vi "OperateDatabase.vi"(8 "error in (no error)":errorcluster, 10 "Person in":refnum<class "Person.lvclass">, 11 "State_Visitor in":refnum<class "State_Visitor.lvclass">) -> (0 "error out":errorcluster, 2 "Person out":refnum<class "Person.lvclass">, 3 "State_Visitor out":refnum<class "State_Visitor.lvclass">)   [LabVIEW 2014, in "State_Visitor.lvclass"]
uses:
  State_Visitor.lvclass
  Person_Class/Person.lvclass
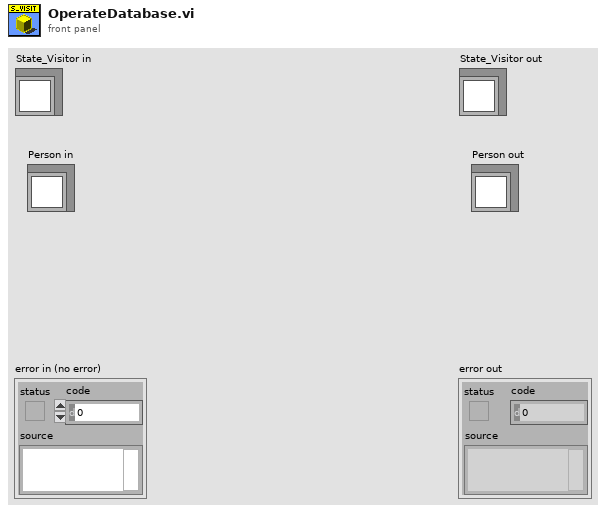
[diagram p1: front panel]
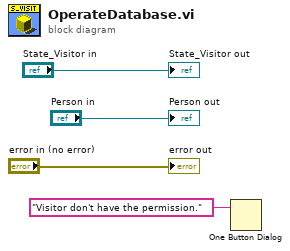
[diagram p0: block diagram]
diagram:
  n1 = One Button Dialog(message="Visitor don't have the permission.") -> ()  [unwired: 1 in, 1 out]
  "error out" <- "error in (no error)"
  "State_Visitor out" <- "State_Visitor in"
  "Person out" <- "Person in"
